vi "Counter_PWMOutput_Test.vi"() -> ()   [LabVIEW 2020]
panel:
  in  "low period(s)":dbl[](array[numeric])=[0.02]
  in  "high period(s)":dbl[](array[numeric])=[0.08]
  out "error out":errorcluster
  in  "stop":bool
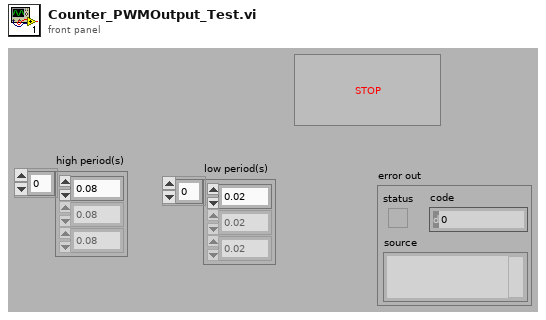
[diagram p1: front panel]
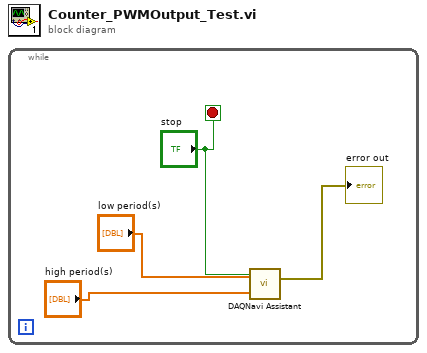
[diagram p0: block diagram]
diagram:
  n1 = while {
    stop <- "stop" stop-if-true
    n2 = call "DAQNavi Assistant"("stop(true)"="stop", "high period(s)"="high period(s)", "low period(s)"="low period(s)") -> ("error out"=→"error out":errorcluster)  [unwired: 2 in, 22 out]
  }
